vi "Adjust Window.vi"(6 "New Bounds":T1 caption="新边界", 7 "Include Paths Ref":refnum<vi> caption="包括路径引用", 8 "Move down Button Ref":refnum<vi> caption="下移按钮引用", 9 "Move up Button Ref":refnum<vi> caption="上移按钮引用", 10 "Remove Button Ref":refnum<vi> caption="删除按钮引用", 11 "New Path Button Ref":refnum<vi> caption="新路径按钮引用") -> ()   [LabVIEW 2011, in "NISAST Include Paths.xctl"]
uses:
  NISAST Include Paths.xctl
  <vilib>/Utility/miscctls.llb/LVRectTypeDef.ctl
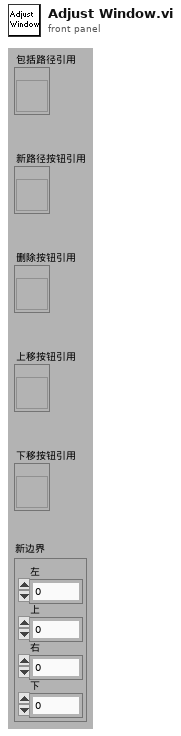
[diagram p1: front panel]
types:
  T1 = typedef "LVRectTypeDef.ctl" = cluster{"Left":i16, "Top":i16, "Right":i16, "Bottom":i16}
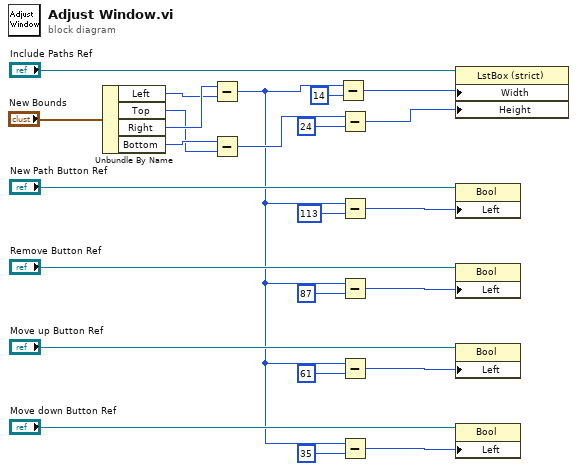
[diagram p0: block diagram]
diagram:
  n1 = Unbundle By Name("New Bounds") -> ("Left"=w20:i16, "Top"=w18:i16, "Right"=w21:i16, "Bottom"=w19:i16)
  n2 = Subtract(x=w21, y=w20) -> (x-y=w2:i16)
  n3 = Subtract(x=w19, y=w18) -> (x-y=w17:i16)
  n4 = Subtract(x=w2, y=u32 14) -> (x-y=w1:u32)
  n5 = Subtract(x=w17, y=u32 24) -> (x-y=w24:u32)
  n6 = Subtract(x=w2, y=u32 113) -> (x-y=w11:u32)
  n7 = Subtract(x=w2, y=u32 87) -> (x-y=w8:u32)
  n8 = Subtract(x=w2, y=u32 61) -> (x-y=w9:u32)
  n9 = Subtract(x=w2, y=u32 35) -> (x-y=w10:u32)
  n10 = property class="LstBox (strict)"(reference="Include Paths Ref", "Width"=w1, "Height"=w24) -> ()  [unwired: 1 in, 2 out]
  n11 = property class="Bool"(reference="New Path Button Ref", "Left"=w11) -> ()  [unwired: 1 in, 2 out]
  n12 = property class="Bool"(reference="Remove Button Ref", "Left"=w8) -> ()  [unwired: 1 in, 2 out]
  n13 = property class="Bool"(reference="Move up Button Ref", "Left"=w9) -> ()  [unwired: 1 in, 2 out]
  n14 = property class="Bool"(reference="Move down Button Ref", "Left"=w10) -> ()  [unwired: 1 in, 2 out]
